vi "Euler 005.vi"() -> ()   [LabVIEW 2025]
uses:
  <vilib>/gmath/NI_AAL_MathFunc.lvlib
panel:
  out "LCM Using Prime Factors":u64
  out "i":i32
  out "i":i32
  out "Slightly better brute force":i32
  out "Brute Force":i32
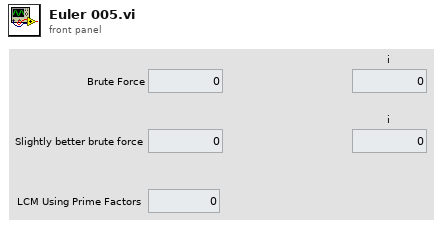
[diagram p1: front panel]
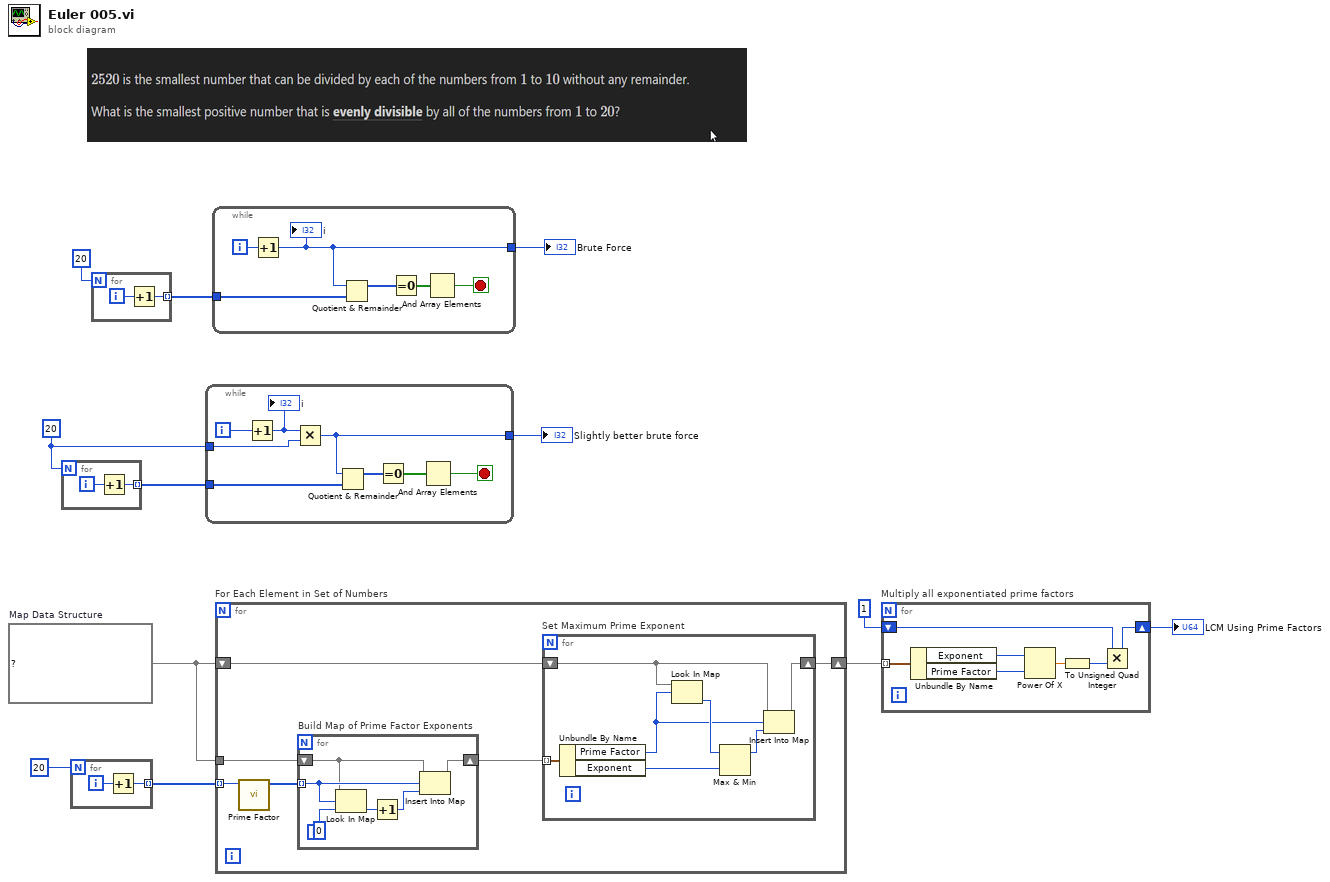
[diagram p0: block diagram]
diagram:
  w5 = 20
  w9 = map{i64, i32} {}  # Map Data Structure
  n1 = for {
    N: w5 -> [_]
    tunnel: [w14] -> w2 mode=indexing
    i -> [w13]
    n2 = Increment(x=w13) -> (x+1=w14:i32)
  }
  n3 = for {
    N: 20 -> [_]
    tunnel: [w16] -> w11 mode=indexing
    i -> [w15]
    n4 = Increment(x=w15) -> (x+1=w16:i32)
  }
  n5 = for {
    N: 20 -> [_]
    tunnel: [w18] -> w6 mode=indexing
    i -> [w17]
    n6 = Increment(x=w17) -> (x+1=w18:i32)
  }
  n7 = while {
    tunnel: w2 -> [w26]
    tunnel: [w21] -> w3
    tunnel: w5 -> [w19]
    i -> [w22]
    stop <- w23 stop-if-true
    n8 = Increment(x=w22) -> (x+1=w20:i32)
    "i" <- w20
    n9 = Multiply(x=w20, y=w19) -> (x*y=w21:i32)
    n10 = Quotient & Remainder(x=w21, y=w26) -> (x-y*floor(x/y)=w25:i32[])  [unwired: 1 out]
    n11 = Equal To 0?(x=w25) -> (x = 0?=w24:bool[])
    n12 = And Array Elements(Boolean array=w24) -> (logical AND=w23:bool)
  }
  "Slightly better brute force" <- w3
  n13 = while {
    tunnel: w6 -> [w32]
    tunnel: [w27] -> w4
    i -> [w28]
    stop <- w29 stop-if-true
    n14 = Increment(x=w28) -> (x+1=w27:i32)
    "i" <- w27
    n15 = Quotient & Remainder(x=w27, y=w32) -> (x-y*floor(x/y)=w31:i32[])  [unwired: 1 out]
    n16 = Equal To 0?(x=w31) -> (x = 0?=w30:bool[])
    n17 = And Array Elements(Boolean array=w30) -> (logical AND=w29:bool)
  }
  "Brute Force" <- w4
  n18 = for "For Each Element in Set of Numbers" {
    tunnel: w11 -> [w38] mode=indexing
    tunnel: w9 -> [w36]
    shift-right: [w35] -> w8
    shift-left: w9 -> [w34]
    n19 = call <vilib>:"Prime Factor.vi"("n"=w38) -> ("Prime Factors"=w37:i64[])  [unwired: 9 in]
    n20 = for "Build Map of Prime Factor Exponents" {
      tunnel: w37 -> [w48] mode=indexing
      shift-right: [w47] -> w33
      shift-left: w36 -> [w46]
      n21 = Look In Map(map=w46, key=w48, default value=0) -> (value=w51:i32)  [unwired: 1 out]
      n22 = Increment(x=w51) -> (x+1=w50:i32)
      n23 = Insert Into Map(map in=w46, key=w48, value=w50) -> (map out=w47:map{i64, i32})  [unwired: 2 out]
    }
    n24 = for "Set Maximum Prime Exponent" {
      tunnel: w33 -> [w45] mode=indexing
      shift-right: [w39] -> w35
      shift-left: w34 -> [w40]
      n25 = Unbundle By Name(w45) -> ("Prime Factor"=w41:i64, "Exponent"=w44:i32)
      n26 = Look In Map(map=w40, key=w41) -> (value=w42:i32)  [unwired: 1 in, 1 out]
      n27 = Max & Min(x=w42, y=w44) -> (max(x,y)=w43:i32)  [unwired: 1 out]
      n28 = Insert Into Map(map in=w40, key=w41, value=w43) -> (map out=w39:map{i64, i32})  [unwired: 2 out]
    }
  }
  n29 = for "Multiply all exponentiated prime factors" {
    tunnel: w8 -> [w54] mode=indexing
    shift-right: [w55] -> w12
    shift-left: u64 1 -> [w56]
    n30 = Unbundle By Name(w54) -> ("Exponent"=w53:i32, "Prime Factor"=w52:i64)
    n31 = Power Of X(1:w52, 2:w53) -> (0:w58:dbl)
    n32 = To Unsigned Quad Integer(1:w58) -> (0:w57:u64)
    n33 = Multiply(x=w56, y=w57) -> (x*y=w55:u64)
  }
  "LCM Using Prime Factors" <- w12
